vi "svfa_Peak to RMS to Peak2Peak.vi"(0 "input signal":dbl[](array[numeric]) format="%.2f", 1 "x-axis units":T1 items=["Time (s)"=0, "Frequency-CB (Hz)"=1, "Frequency-CPB (Hz)"=1248, "Frequency-Arbitrary (Hz)"=2357, "Quefrency (s)"=2, "Revolutions (rev)"=3, "Order"=4, "Speed (RPM)"=11, "Speed (rad/s)"=21, "Critical Band"=31, "Critical Band Rate (Bark)"=32, "Index"=65535], 2 "x0":dbl format="%.2f", 3 "view desired":enum16{"no change", "rms", "peak", "peak-peak"}(ring), 5 "linear/dB":enum16{"linear", "dB"}(ring), 7 "power/magnitude":enum16{"power", "magnitude"}(ring), 9 "view in":enum16{"rms", "peak", "peak-peak"}(ring), 11 "dB reference":dbl format="%.2f") -> (4 "scale converted signal":dbl[](array[numeric]) format="%.2f", 6 "linear/dB (dupl)":enum16{"linear", "dB"}(ring), 8 "power/magnitude (dupl)":enum16{"power", "magnitude"}(ring), 10 "view out":enum16{"rms", "peak", "peak-peak"}(ring), 15 "dB reference (dupl)":dbl format="%.2f")   [LabVIEW 2017]
doc: "This VI should only be used when the array is bandlimited in the sense that there is a known relationship between rms, peak, and peak to peak levels.\n\nFor instance, for an FFT spectrum, each bin represents a unique-frequency tone where it is known that 0.7071 EU rms = 1 EU pk = 2 EU pk-pk\n\nGeneral time signals are not bandlimited and there is no fixed ratio between peak units which is why crest factor is measured for generic broadband signals."
uses:
  <vilib>/addons/_NISVFA/_Shared subVIs/Controls/svc_X-Axis Units.ctl
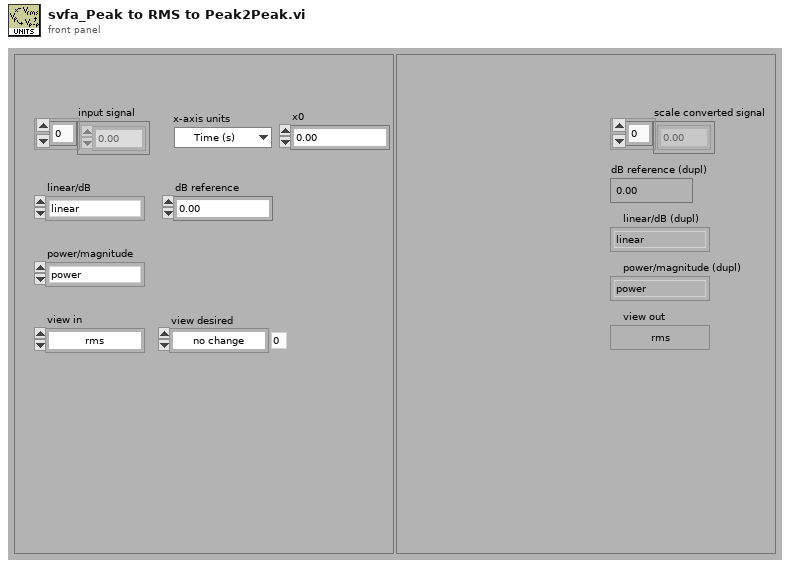
[diagram p1: front panel]
types:
  T1 = typedef "svc_X-Axis Units.ctl" = u16
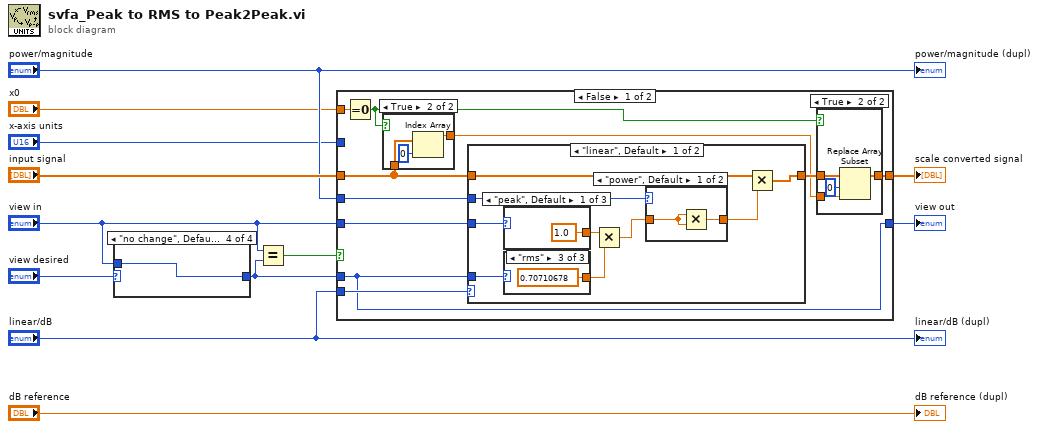
[diagram p0: block diagram]
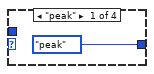
[diagram p2: hidden frame]
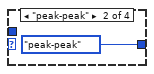
[diagram p3: hidden frame]
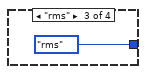
[diagram p4: hidden frame]
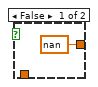
[diagram p6: hidden frame]
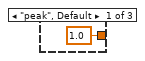
[diagram p8: hidden frame]
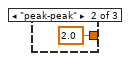
[diagram p9: hidden frame]
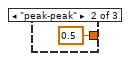
[diagram p10: hidden frame]
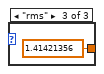
[diagram p11: hidden frame]
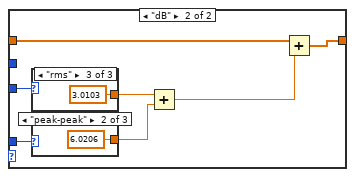
[diagram p12: hidden frame]
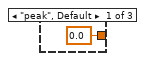
[diagram p13: hidden frame]
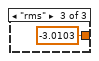
[diagram p14: hidden frame]
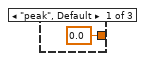
[diagram p15: hidden frame]
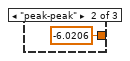
[diagram p16: hidden frame]
diagram:
  n1 = case shown="\"no change\", Default" "view desired" {
    tunnel: [enum16{"rms", "peak", "peak-peak"}."peak" ("view in") enum16{"rms", "peak", "peak-peak"}."peak-peak" ("view in") enum16{"rms", "peak", "peak-peak"}."rms" ("view in") w16] -> w4
    tunnel: "view in" -> [_ _ _ w16]
    frame "peak" {
    }
    frame "peak-peak" {
    }
    frame "rms" {
    }
    frame "no change", Default {
    }
  }
  n2 = Equal?(x="view in", y=w4) -> (x = y?=w3:bool)
  n3 = case shown="False" w3 {
    tunnel: [w18 w68] -> w12
    tunnel: w4 -> [w23 _]
    tunnel: "input signal" -> [w21 w68]
    tunnel: "linear/dB" -> [w25 _]
    tunnel: "power/magnitude" -> [w24 _]
    tunnel: "view in" -> [w26 w67]
    tunnel: [w23 w67] -> w8
    tunnel: "x0" -> [w22 _]
    tunnel: "x-axis units" -> [_ _]
    frame False {
      n4 = Equal To 0?(x=w22) -> (x = 0?=w17:bool)
      n5 = case shown="True" w17 {
        tunnel: w21 -> [_ w35]
        tunnel: [nan ("dB reference") w33] -> w19
        frame False {
        }
        frame True {
          n6 = Index Array(array=w35, index=0 ("Index")) -> (element=w33:dbl)
        }
      }
      n7 = case shown="\"linear\", Default" w25 {
        tunnel: w23 -> [w40 w58]
        tunnel: [w39 w59] -> w20
        tunnel: w24 -> [w38 _]
        tunnel: w26 -> [w42 w54]
        tunnel: w21 -> [w41 w60]
        frame "linear", Default {
          n8 = case shown="\"peak\", Default" w42 {
            tunnel: [1.0 ("y") 0.5 ("y") 1.41421356 ("y")] -> w44
            frame "peak", Default {
            }
            frame "peak-peak" {
            }
            frame "rms" {
            }
          }
          n9 = case shown="\"rms\"" w40 {
            tunnel: [1.0 ("y") 2.0 ("y") 0.70710678 ("y")] -> w43
            frame "peak", Default {
            }
            frame "peak-peak" {
            }
            frame "rms" {
            }
          }
          n10 = Multiply(x=w44, y=w43) -> (x*y=w37:dbl)
          n11 = case shown="\"power\", Default" w38 {
            tunnel: w37 -> [w46 w47]
            tunnel: [w45 w47] -> w36
            frame "power", Default {
              n12 = Multiply(x=w46, y=w46) -> (x*y=w45:dbl)
            }
            frame "magnitude" {
            }
          }
          n13 = Multiply(x=w41, y=w36) -> (x*y=w39:dbl[])
        }
        frame "dB" {
          n14 = case shown="\"rms\"" w54 {
            tunnel: [0.0 ("y") -6.0206 ("y") 3.0103 ("y")] -> w57
            frame "peak", Default {
            }
            frame "peak-peak" {
            }
            frame "rms" {
            }
          }
          n15 = case shown="\"peak-peak\"" w58 {
            tunnel: [0.0 ("y") 6.0206 ("y") -3.0103 ("y")] -> w56
            frame "peak", Default {
            }
            frame "peak-peak" {
            }
            frame "rms" {
            }
          }
          n16 = Add(x=w57, y=w56) -> (x+y=w55:dbl)
          n17 = Add(x=w60, y=w55) -> (x+y=w59:dbl[])
        }
      }
      n18 = case shown="True" w17 {
        tunnel: w20 -> [w27 w31]
        tunnel: w19 -> [_ w29]
        tunnel: [w27 w28] -> w18
        frame False {
        }
        frame True {
          n19 = Replace Array Subset(array=w31, new element=w29, index=0 ("Index")) -> (w28:dbl[])
        }
      }
    }
    frame True {
    }
  }
  "view out" <- w8
  "scale converted signal" <- w12
  "linear/dB (dupl)" <- "linear/dB"
  "power/magnitude (dupl)" <- "power/magnitude"
  "dB reference (dupl)" <- "dB reference"
